vi "DIO - Enable Digital Input.vi"(8 "error in":errorcluster, 10 "Channel Number":i32, 11 "TCP Network Connection in":refnum<k5>) -> (0 "error out":errorcluster, 3 "TCP Network Connection out":refnum<k5>)   [LabVIEW 2020]
doc: "Enables the DIO port, and sets the digital line to be an input."
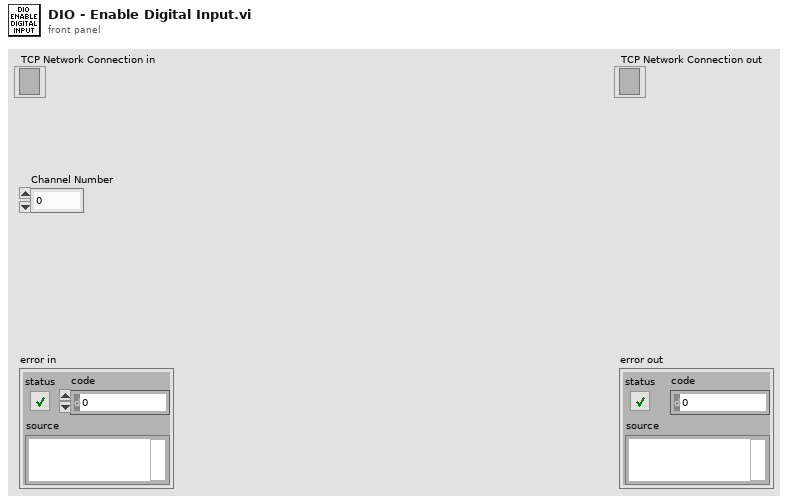
[diagram p1: front panel]
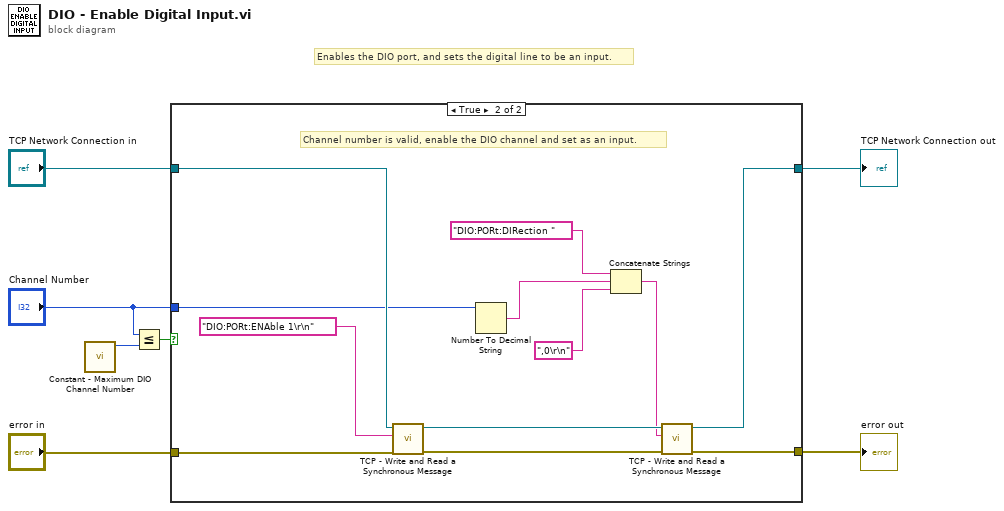
[diagram p0: block diagram]
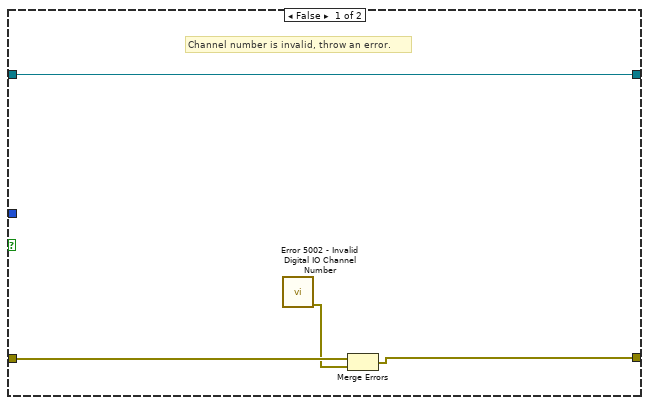
[diagram p2: hidden frame]
diagram:
  # "Enables the DIO port, and sets the digital line to be an input."
  n1 = call "Constant - Maximum DIO Channel Number.vi"() -> ("Maximum Channel"=w2:i32)  [unwired: 11 in]
  n2 = Less Or Equal?(x="Channel Number", y=w2) -> (x <= y?=w1:bool)
  n3 = case shown="True" w1 {
    tunnel: "error in" -> [w10 w23]
    tunnel: "TCP Network Connection in" -> [w11 w22]
    tunnel: [w8 w18] -> w5
    tunnel: [w11 w13] -> w4
    tunnel: "Channel Number" -> [_ w12]
    frame False {
      # "Channel number is invalid, throw an error."
      n4 = call "Error 5002 - Invalid Digital IO Channel Number.vi"() -> ("error out"=w9:errorcluster)  [unwired: 11 in]
      n5 = Merge Errors(w10, w9) -> (w8:errorcluster)
    }
    frame True {
      # "Channel number is valid, enable the DIO channel and set as an input."
      n6 = call "TCP - Write and Read a Synchronous Message.vi"("error in"=w23, "Message to Send"="DIO:PORt:ENAble 1\r\n", "TCP Network Connection in"=w22) -> ("error out"=w19:errorcluster, "TCP Network Connection out"=w20:refnum<k5>)  [unwired: 6 in, 1 out]
      n7 = Number To Decimal String(number=w12) -> (decimal integer string=w15:string)  [unwired: 1 in]
      n8 = Concatenate Strings("DIO:PORt:DIRection " ("Message to Send"), w15, ",0\r\n" ("string")) -> (w16:string)
      n9 = call "TCP - Write and Read a Synchronous Message.vi"("error in"=w19, "Message to Send"=w16, "TCP Network Connection in"=w20) -> ("error out"=w18:errorcluster, "TCP Network Connection out"=w13:refnum<k5>)  [unwired: 6 in, 1 out]
    }
  }
  "TCP Network Connection out" <- w4
  "error out" <- w5
